vi "test1-ProcessSyncMessageInCSMLoop(SendAndReceive).vi"(8 "error in (no error)":errorcluster, 11 "TestCase in":refnum<class "testcase-CSMAddonLoopSupport.lvclass">) -> (0 "error out":errorcluster, 3 "TestCase out":refnum<class "testcase-CSMAddonLoopSupport.lvclass">)   [LabVIEW 2017, in "testcase-CSMAddonLoopSupport.lvclass"]
uses:
  testcase-CSMAddonLoopSupport.lvclass
  4585ddd5-ba69-4fd4-94fe-207595864cbd.vi
  a7620e19-6451-46a1-85ca-ade5edb58587.vi
  55fec5d7-cd22-46f7-b641-2c7c49619fc8.vi
  9cfd6824-310a-46c9-9b98-3854de5c7aa2.vi
  <vilib>/addons/_JKI Toolkits/VI Tester/TestCase.llb/TestCase.lvclass
  src/user.lib/_NEVSTOP/Communicable State Machine(CSM)/Communicable State Machine.lvlib
  C:/Program Files (x86)/National Instruments/LabVIEW 2017/vi.lib/addons/_JKI Toolkits/VI Tester/TestCase.llb/TestCase.lvclass
panel:
  out "LoopCount":i32
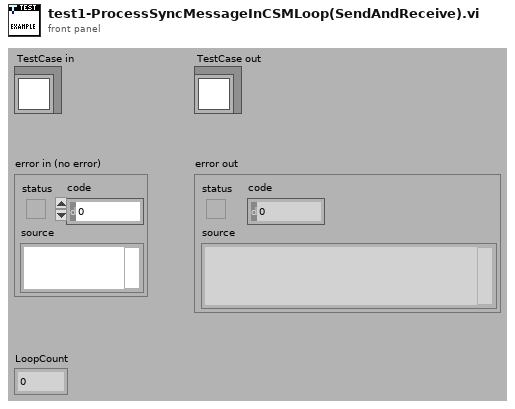
[diagram p1: front panel]
types:
  T1 = cluster{"Arguments":string, "Response":string, "error":errorcluster}
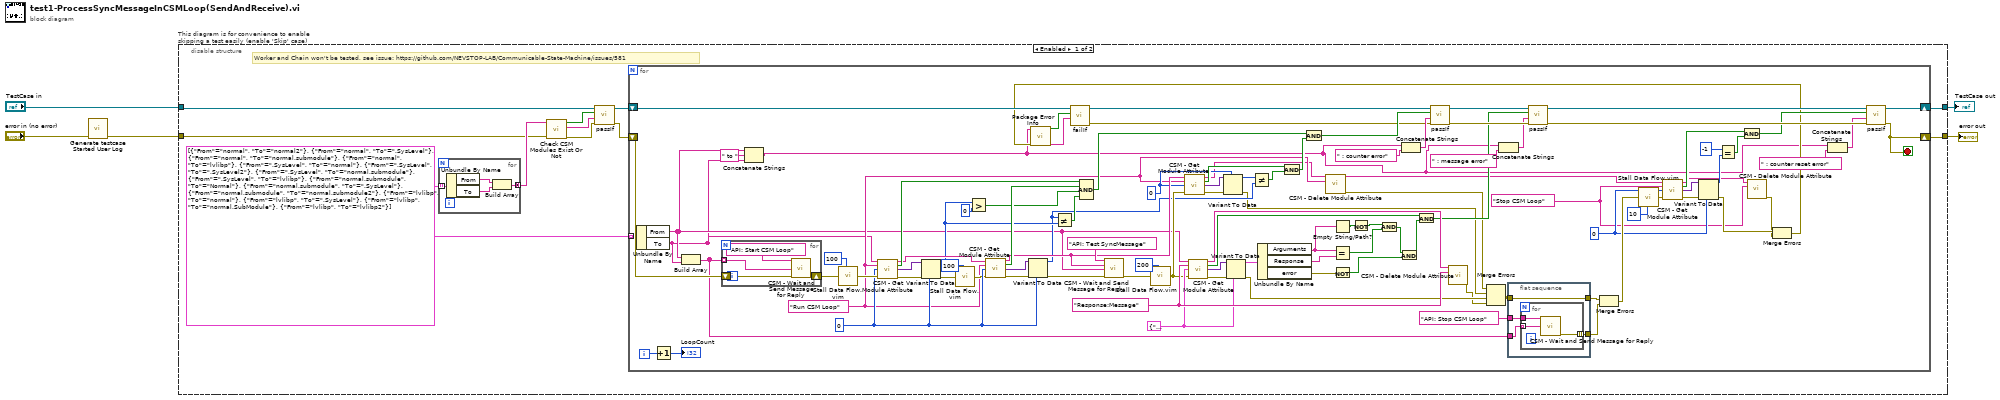
[diagram p0: block diagram]
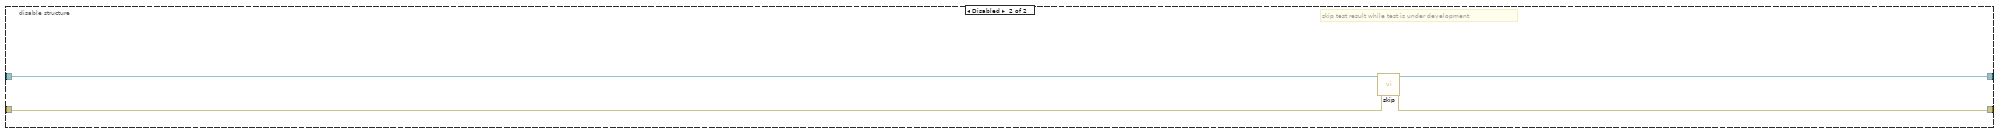
[diagram p2: hidden frame]
diagram:
  n1 = call "Generate testcase Started User Log.vi"("Error In"="error in (no error)") -> ("error out"=w1:errorcluster)  [unwired: 10 in]
  n2 = disable-structure "This diagram is for convenience to enable skipping a test easily (enable 'Skip' case)" shown="Enabled" {
    disable-tunnel: "TestCase in" -> [w13 w139]
    disable-tunnel: [w16 w137] -> w2
    disable-tunnel: [w15 w138] -> w4
    disable-tunnel: w1 -> [w6 w136]
    frame Enabled {
      w10 = cluster{"From":string, "To":string}[] [{"From"="normal", "To"="normal2"}, {"From"="normal", "To"=".SysLevel"}, {"From"="normal", "To"="normal.submodule"}, {"From"="normal", "To"="lvlibp"}, {"From"=".SysLevel", "To"="normal"}, {"From"=".SysLevel", "To"=".SysLevel2"}, {"From"=".SysLevel", "To"="normal.submodule"}, {"From"=".SysLevel", "To"="lvlibp"}, {"From"="normal.submodule", "To"="Normal"}, {"From"="normal.submodule", "To"=".SysLevel"}, {"From"="normal.submodule", "To"="normal.submodule2"}, {"From"="lvlibp", "To"="normal"}, {"From"="lvlibp", "To"=".SysLevel"}, {"From"="lvlibp", "To"="normal.SubModule"}, {"From"="lvlibp", "To"="lvlibp2"}]
      # "Worker and Chain won't be tested, see issue: https://github.com/NEVSTOP-LAB/Communicable-State-Machine/issues/581"
      n3 = for {
        tunnel: w10 -> [w20] mode=indexing
        tunnel: [w17] -> w9 mode=concatenating
        n4 = Unbundle By Name(w20) -> ("From"=w19:string, "To"=w18:string)
        n5 = Build Array(w19, w18) -> (w17:string[])
      }
      n6 = call "Check CSM Modules Exist Or Not.vi"("error in"=w6, "CSM names in"=w9) -> ("error out"=w7:errorcluster, "Debug string"=w8:string, "All Modules Exist?"=w14:bool)  [unwired: 7 in]
      n7 = call-dynamic "passIf.vi"("error in (no error)"=w7, "message (\"\")"=w8, "pass"=w14, "TestCase in"=w13) -> ("error out"=w11:errorcluster, "TestCase out"=w12:refnum<class "testcase-CSMAddonLoopSupport.lvclass">)  [unwired: 6 in]
      n8 = for {
        tunnel: w10 -> [w40] mode=indexing
        shift-right: [w29] -> w16
        shift-left: w12 -> [w25]
        shift-right: [w28] -> w15
        shift-left: w11 -> [w66]
        i -> [w124]
        stop <- w28 stop-if-true
        w43 = "Stop CSM Loop" ("State")
        w56 = 0
        w76 = 0
        w91 = 0
        w47 = "Run CSM Loop" ("State")
        w102 = T1 {"Arguments"="", "Response"="", "error"={"status"=FALSE, "code"=0, "source"=""}}
        w103 = "Response:Message" ("State")
        n9 = Unbundle By Name(w40) -> ("From"=w38:string, "To"=w37:string)
        n10 = Increment(x=w124) -> (x+1=→"LoopCount":i32)
        n11 = Build Array(w38, w37) -> (w39:string[])
        n12 = for {
          shift-right: [w127] -> w122
          shift-left: w66 -> [w126]
          tunnel: w39 -> [w125] mode=indexing
          n13 = call "CSM - Wait and Send Message for Reply.vi"("State"="API: Start CSM Loop", "Target Module"=w125, "Error In (No Error)"=w126) -> ("error out"=w127:errorcluster)  [unwired: 9 in, 3 out]
        }
        n14 = Concatenate Strings(w38, " to " ("string"), w37) -> (w21:string)
        n15 = call "Stall Data Flow.vim"("value in"=w122, "milliseconds to wait"=u32 100) -> ("value out"=w99:errorcluster)  [unwired: 1 out]
        n16 = call "CSM - Get Module Attribute.vi"("CSM Name"=w37, "Attribute"=w47, "Default Value (Empty Variant)"=w91, "Error In"=w99) -> ("CSM Name (Dup)"=w93:string, "Found"=w98:bool, "Value"=w92:variant, "error out"=w96:errorcluster)  [unwired: 7 in, 1 out]
        n17 = Variant To Data(error in=w96, type=w91, Variant=w92) -> (data=w86:i32, error out=w85:errorcluster)
        n18 = call "Stall Data Flow.vim"("value in"=w85, "milliseconds to wait"=u32 100) -> ("value out"=w84:errorcluster)  [unwired: 1 out]
        n19 = Greater?(x=w86, y=0) -> (0:w89:bool)
        n20 = call "CSM - Get Module Attribute.vi"("CSM Name"=w93, "Attribute"=w47, "Default Value (Empty Variant)"=w91, "Error In"=w84) -> ("CSM Name (Dup)"=w81:string, "Found"=w97:bool, "Value"=w88:variant, "error out"=w95:errorcluster)  [unwired: 7 in, 1 out]
        n21 = Variant To Data(error in=w95, type=w91, Variant=w88) -> (data=w74:i32, error out=w94:errorcluster)
        n22 = Not Equal?(x=w74, y=w86) -> (x != y?=w87:bool)
        n23 = Compound Arithmetic op=AND(w98, w97, w89, w87) -> (w73:bool)
        n24 = call "CSM - Wait and Send Message for Reply.vi"("State"="API: Test SyncMessage", "Arguments (\"\")"=w81, "Target Module"=w38, "Error In (No Error)"=w94) -> ("error out"=w118:errorcluster)  [unwired: 8 in, 3 out]
        n25 = call "Stall Data Flow.vim"("value in"=w118, "milliseconds to wait"=u32 200) -> ("value out"=w82:errorcluster)  [unwired: 1 out]
        n26 = call "CSM - Get Module Attribute.vi"("CSM Name"=w81, "Attribute"=w47, "Default Value (Empty Variant)"=w76, "Error In"=w82) -> ("CSM Name (Dup)"=w46:string, "Found"=w78:bool, "Value"=w77:variant, "error out"=w79:errorcluster)  [unwired: 7 in, 1 out]
        n27 = call "CSM - Get Module Attribute.vi"("CSM Name"=w38, "Attribute"=w103, "Default Value (Empty Variant)"=w102, "Error In"=w82) -> ("CSM Name (Dup)"=w111:string, "Found"=w113:bool, "Value"=w116:variant, "error out"=w117:errorcluster)  [unwired: 7 in, 1 out]
        n28 = Variant To Data(error in=w79, type=w76, Variant=w77) -> (data=w75:i32, error out=w45:errorcluster)
        n29 = Variant To Data(error in=w117, type=w102, Variant=w116) -> (data=w115:T1, error out=w101:errorcluster)
        n30 = Not Equal?(x=w75, y=w74) -> (x != y?=w80:bool)
        n31 = Unbundle By Name(w115) -> ("Arguments"=w106:string, "Response"=w105:string, "error"=w104:errorcluster)
        n32 = Compound Arithmetic op=AND(w78, w80) -> (w72:bool)
        n33 = And(x=w73, y=w72) -> (x .and. y?=w71:bool)
        n34 = call "CSM - Delete Module Attribute.vi"("CSM Name"=w46, "Attribute"=w47) -> ("CSM Name (Dup)"=w42:string, "error out"=w44:errorcluster)  [unwired: 10 in, 2 out]
        n35 = Empty String/Path?(string/path=w106) -> (empty?=w110:bool)
        n36 = Equal?(x=w106, y=w105) -> (x = y?=w108:bool)
        n37 = Not(x=w104) -> (.not. x?=w114:bool)
        n38 = Not(x=w110) -> (.not. x?=w109:bool)
        n39 = And(x=w109, y=w108) -> (x .and. y?=w107:bool)
        n40 = And(x=w107, y=w114) -> (x .and. y?=w112:bool)
        n41 = Concatenate Strings(w21, " : counter error" ("format string")) -> (w34:string)
        n42 = And(x=w113, y=w112) -> (x .and. y?=w68:bool)
        n43 = call "CSM - Delete Module Attribute.vi"("CSM Name"=w111, "Attribute"=w103) -> ("error out"=w100:errorcluster)  [unwired: 10 in, 3 out]
        n44 = Merge Errors(w44, w45, w101, w100) -> (w48:errorcluster)
        n45 = Concatenate Strings(w21, " : message error" ("format string")) -> (w32:string)
        n46 = flat-sequence {
          tunnel: "API: Stop CSM Loop" ("State") -> [w132]
          tunnel: [w131] -> w63
          tunnel: [w130] -> w49
          tunnel: w48 -> [w130]
          tunnel: w39 -> [w129]
          frame #0 {
            n47 = for {
              tunnel: w132 -> [w135]
              tunnel: [w134] -> w131 mode=indexing
              tunnel: w129 -> [w133] mode=indexing
              n48 = call "CSM - Wait and Send Message for Reply.vi"("State"=w135, "Target Module"=w133) -> ("error out"=w134:errorcluster)  [unwired: 10 in, 3 out]
            }
          }
        }
        n49 = Merge Errors(w49, w63) -> (w61:errorcluster)
        n50 = call "Stall Data Flow.vim"("value in"=w61, "milliseconds to wait"=u32 10) -> ("value out"=w60:errorcluster)  [unwired: 1 out]
        n51 = call "CSM - Get Module Attribute.vi"("CSM Name"=w42, "Attribute"=w43, "Default Value (Empty Variant)"=w56, "Error In"=w60) -> ("CSM Name (Dup)"=w41:string, "Found"=w59:bool, "Value"=w57:variant, "error out"=w58:errorcluster)  [unwired: 7 in, 1 out]
        n52 = Variant To Data(error in=w58, type=w56, Variant=w57) -> (data=w55:i32, error out=w51:errorcluster)
        n53 = Equal?(x=-1, y=w55) -> (x = y?=w52:bool)
        n54 = And(x=w59, y=w52) -> (x .and. y?=w53:bool)
        n55 = call "CSM - Delete Module Attribute.vi"("CSM Name"=w41, "Attribute"=w43) -> ("error out"=w50:errorcluster)  [unwired: 10 in, 3 out]
        n56 = Merge Errors(w51, w50) -> (w22:errorcluster)
        n57 = call "Package Error Info.vi"("error in"=w22, "String in"=w21) -> ("packed error info out"=w26:string, "error status"=w27:bool)  [unwired: 8 in]
        n58 = call-dynamic "failIf.vi"("message (\"\")"=w26, "fail"=w27, "TestCase in"=w25) -> ("error out"=w23:errorcluster, "TestCase out"=w24:refnum<class "testcase-CSMAddonLoopSupport.lvclass">)  [unwired: 7 in]
        n59 = call-dynamic "passIf.vi"("error in (no error)"=w23, "message (\"\")"=w34, "pass"=w71, "TestCase in"=w24) -> ("error out"=w69:errorcluster, "TestCase out"=w70:refnum<class "testcase-CSMAddonLoopSupport.lvclass">)  [unwired: 6 in]
        n60 = call-dynamic "passIf.vi"("error in (no error)"=w69, "message (\"\")"=w32, "pass"=w68, "TestCase in"=w70) -> ("error out"=w64:errorcluster, "TestCase out"=w65:refnum<class "testcase-CSMAddonLoopSupport.lvclass">)  [unwired: 6 in]
        n61 = Concatenate Strings(w21, " : counter reset error" ("format string")) -> (w30:string)
        n62 = call-dynamic "passIf.vi"("error in (no error)"=w64, "message (\"\")"=w30, "pass"=w53, "TestCase in"=w65) -> ("error out"=w28:errorcluster, "TestCase out"=w29:refnum<class "testcase-CSMAddonLoopSupport.lvclass">)  [unwired: 6 in]
      }
    }
    frame Disabled {
      # "skip test result while test is under development"
      n63 = call <vilib>:"skip.vi"("error in (no error)"=w136, "TestCase in"=w139) -> ("error out"=w138:errorcluster, "TestCase out"=w137:refnum<class "testcase-CSMAddonLoopSupport.lvclass">)  [unwired: 8 in]
    }
  }
  "error out" <- w4
  "TestCase out" <- w2
